vi "Chalk.vi"(8 "error in (no error)":errorcluster, 10 "Text":string, 11 "Chalk_Control":T1) -> (0 "error out":errorcluster, 3 "Stdout_Text":string)   [LabVIEW 2018, in "CLI.lvclass"]
doc: "Creates ANSI escape codes for FG, BG & Underline settings"
uses:
  CLI.lvclass
  Chalk_Options.ctl
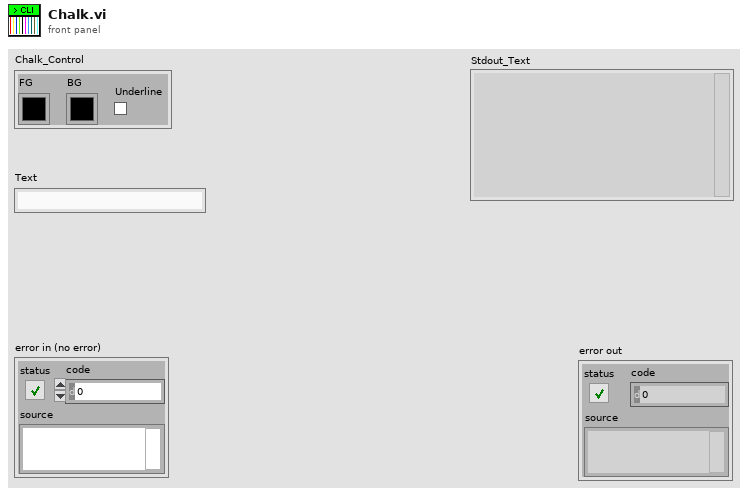
[diagram p1: front panel]
types:
  T1 = typedef "CLI.lvclass/Chalk_Options.ctl" = cluster{"FG":u32, "BG":u32, "Underline":bool}
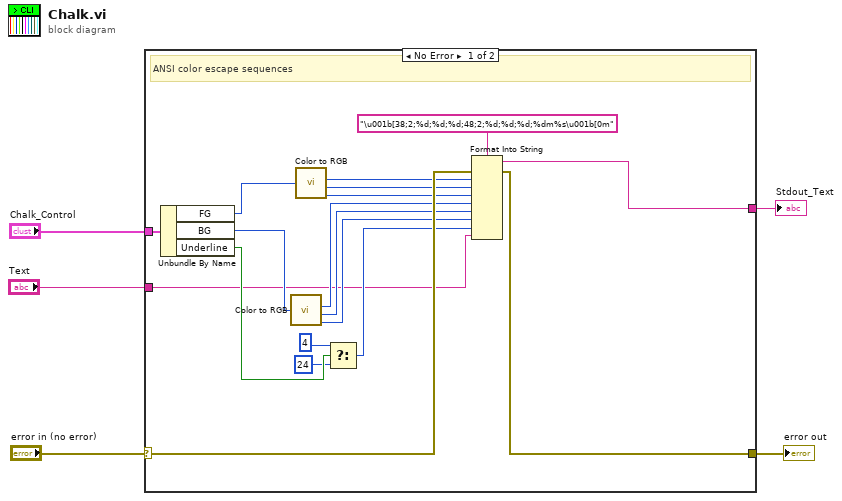
[diagram p0: block diagram]
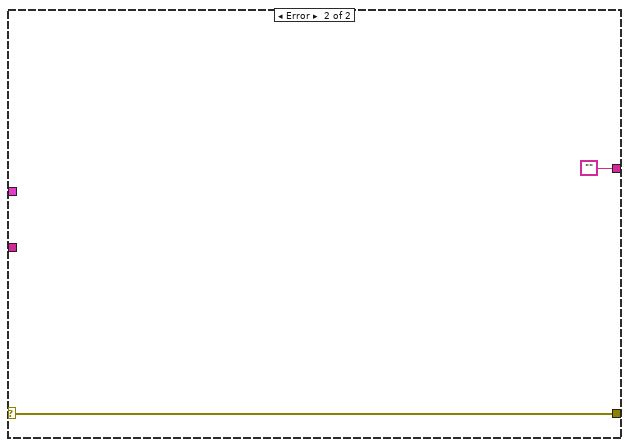
[diagram p2: hidden frame]
diagram:
  n1 = case shown="No Error" "error in (no error)" {
    selector: "error in (no error)" -> [w22 w25]
    tunnel: "Chalk_Control" -> [w20 _]
    tunnel: "Text" -> [w7 _]
    tunnel: [w23 w25] -> w2
    tunnel: [w6 ""] -> w1
    frame No Error {
      # "ANSI color escape sequences"
      n2 = Unbundle By Name(w20) -> ("FG"=w19:u32, "BG"=w15:u32, "Underline"=w11:bool)
      n3 = call <vilib>:"Color to RGB.vi"("Color"=w15) -> ("R"=w14:u8, "G"=w13:u8, "B"=w12:u8)  [unwired: 1 out]
      n4 = call <vilib>:"Color to RGB.vi"("Color"=w19) -> ("R"=w18:u8, "G"=w17:u8, "B"=w16:u8)  [unwired: 1 out]
      n5 = Select(t=u8 4, s=w11, f=u8 24) -> (s? t:f=w8:u8)
      n6 = Format Into String(format string="\u001b[38;2;%d;%d;%d;48;2;%d;%d;%d;%dm%s\u001b[0m", error in=w22, w18, w17, w16, w14, w13, w12, w8, w7) -> (resulting string=w6:string, error out=w23:errorcluster)  [unwired: 1 in]
    }
    frame Error {
    }
  }
  "error out" <- w2
  "Stdout_Text" <- w1
